vi "NewConnection.vi"(8 "error in (no error)":errorcluster caption="エラー入力（エラーなし）", 11 "accesskey":string) -> (0 "error out":errorcluster, 3 "Handler out":T1)   [LabVIEW 2015, in "LV_CloudTranslationAPI.lvlib"]
uses:
  LV_CloudTranslationAPI.lvlib
  Handler.ctl
  <vilib>/httpClient/ClientHandle.ctl
  <vilib>/httpClient/LabVIEWHTTPClient.lvlib
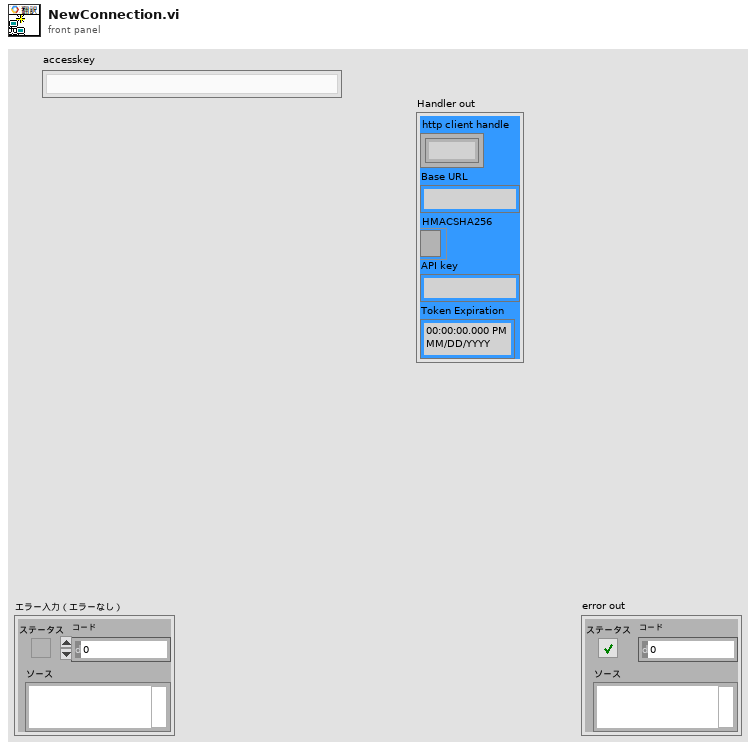
[diagram p1: front panel]
types:
  T1 = typedef "LV_CloudTranslationAPI.lvlib/Handler.ctl" = cluster{"http client handle":T2, "Base URL":string, "HMACSHA256":refnum<k24>, "API key":string, "Token Expiration ":timestamp}
  T2 = typedef "LabVIEWHTTPClient.lvlib/ClientHandle.ctl" = refnum<k1>
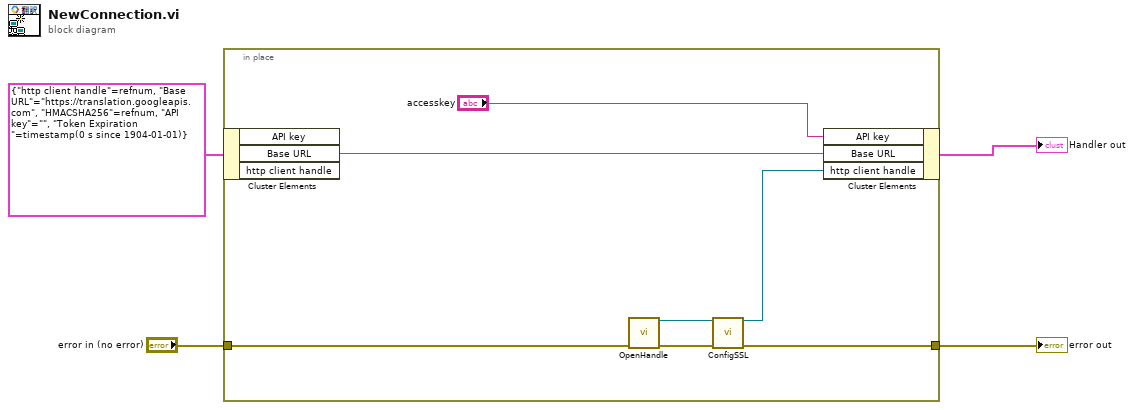
[diagram p0: block diagram]
diagram:
  n1 = in-place {
    in-place-border: [w5] -> w2
    in-place-border: "error in (no error)" -> [w10]
    n2 = in-place-cluster #1(T1 {"http client handle"=refnum, "Base URL"="https://translation.googleapis.com", "HMACSHA256"=refnum, "API key"="", "Token Expiration "=timestamp(0 s since 1904-01-01)} ("Handler in")) -> ("Base URL"=w11:string)  [unwired: 2 out]
    n3 = call <vilib>:"OpenHandle.vi"("error in (no error)"=w10) -> ("client handle out"=w8:T2, "error out"=w6:errorcluster)  [unwired: 13 in]
    n4 = call <vilib>:"ConfigSSL.vi"("client handle"=w8, "error in (no error)"=w6) -> ("client handle out"=w7:T2, "error out"=w5:errorcluster)  [unwired: 12 in]
    n5 = in-place-cluster #1("API key"="accesskey", "Base URL"=w11, "http client handle"=w7) -> (→"Handler out":T1)
  }
  "error out" <- w2
